vi "Switch laser on-off.vi"(9 "Laser On/Off":bool, 11 "VISA resource name":refnum<visa-resource-name>) -> (3 "VISA resource name out":refnum<visa-resource-name>)   [LabVIEW 2017]
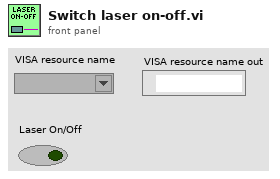
[diagram p1: front panel]
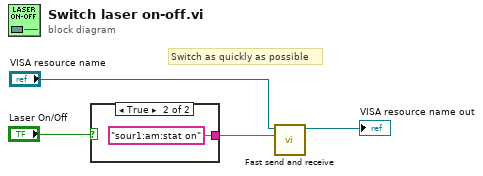
[diagram p0: block diagram]
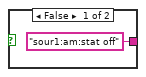
[diagram p2: hidden frame]
diagram:
  # "Switch as quickly as possible"
  n1 = case shown="True" "Laser On/Off" {
    tunnel: ["sour1:am:stat off" "sour1:am:stat on"] -> w2
    frame False {
    }
    frame True {
    }
  }
  n2 = call "Fast send and receive.vi"("write to laser"=w2, "VISA resource name"="VISA resource name") -> ("VISA resource name out"=→"VISA resource name out":refnum<visa-resource-name>)  [unwired: 8 in, 1 out]
